vi "Corrupt DLC.vi"(8 "error in (no error)":errorcluster, 9 "Engine Run-Time Data Cluster In":T1 {"Compiled Data"."Corruption Info DUT_Network"."Frame Infos Array"."CRC Index" min=-7 max=7; "Compiled Data"."Corruption Info DUT_Network"."Frame Infos Array"."DLC Length  Corruption Index" min=-8 max=8; "Compiled Data"."Corruption Info Network_DUT"."Frame Infos Array"."CRC Index" min=-7 max=7; "Compiled Data"."Corruption Info Network_DUT"."Frame Infos Array"."DLC Length  Corruption Index" min=-8 max=8; "Specified Channel Ref List Out" format="%.0x"; "Specified Channel Ref List In" format="%.0x"}, 10 "Frame Infos":T6 {"CRC Index" min=-7 max=7; "DLC Length  Corruption Index" min=-8 max=8}, 11 "CAN frame in":T8 {"payload" format="%x"; "timestamp" format="%<%.7X\n%x>T"; "type" items=["CAN Data"=0, "CAN Remote"=1, "CAN Bus Error"=2, "CAN 2.0 Data"=8, "CAN FD Data"=16, "CAN FD+BRS Data"=24, "J1939 Data"=192, "Delay"=224, "Log Trigger"=225, "Start Trigger"=226]; "identifier" format="%x"}) -> (0 "error out":errorcluster, 3 "CAN frame out":T8 {"payload" format="%x"; "timestamp" format="%<%.7X\n%x>T"; "type" items=["CAN Data"=0, "CAN Remote"=1, "CAN Bus Error"=2, "CAN 2.0 Data"=8, "CAN FD Data"=16, "CAN FD+BRS Data"=24, "J1939 Data"=192, "Delay"=224, "Log Trigger"=225, "Start Trigger"=226]; "identifier" format="%x"})   [LabVIEW 2018, in "CAN Gateway Engine.lvlib"]
uses:
  CAN Gateway Engine.lvlib
  <vilib>/xnet/xnet.llb/XNET Frame CAN.ctl
  <vilib>/xnet/xnet.llb/XNET Frame Type CAN.ctl
  Shared/CTLs/Frame.ctl
  Shared/CTLs/Signal_Data_Trigger.ctl
  Shared/CTLs/Runtime engine Data.ctl
  <vilib>/NI Veristand/Custom Device API/Custom Device Engine Event Ref.ctl
  <vilib>/NI Veristand/Custom Device API/Custom Device Item Ref.ctl
  Shared/CTLs/Compiled Data.ctl
  Shared/CTLs/Corruption Info.ctl
  Shared/CAN Gateway Shared.lvlib
  <vilib>/NI Veristand/Custom Device API/Custom Device API.lvlib
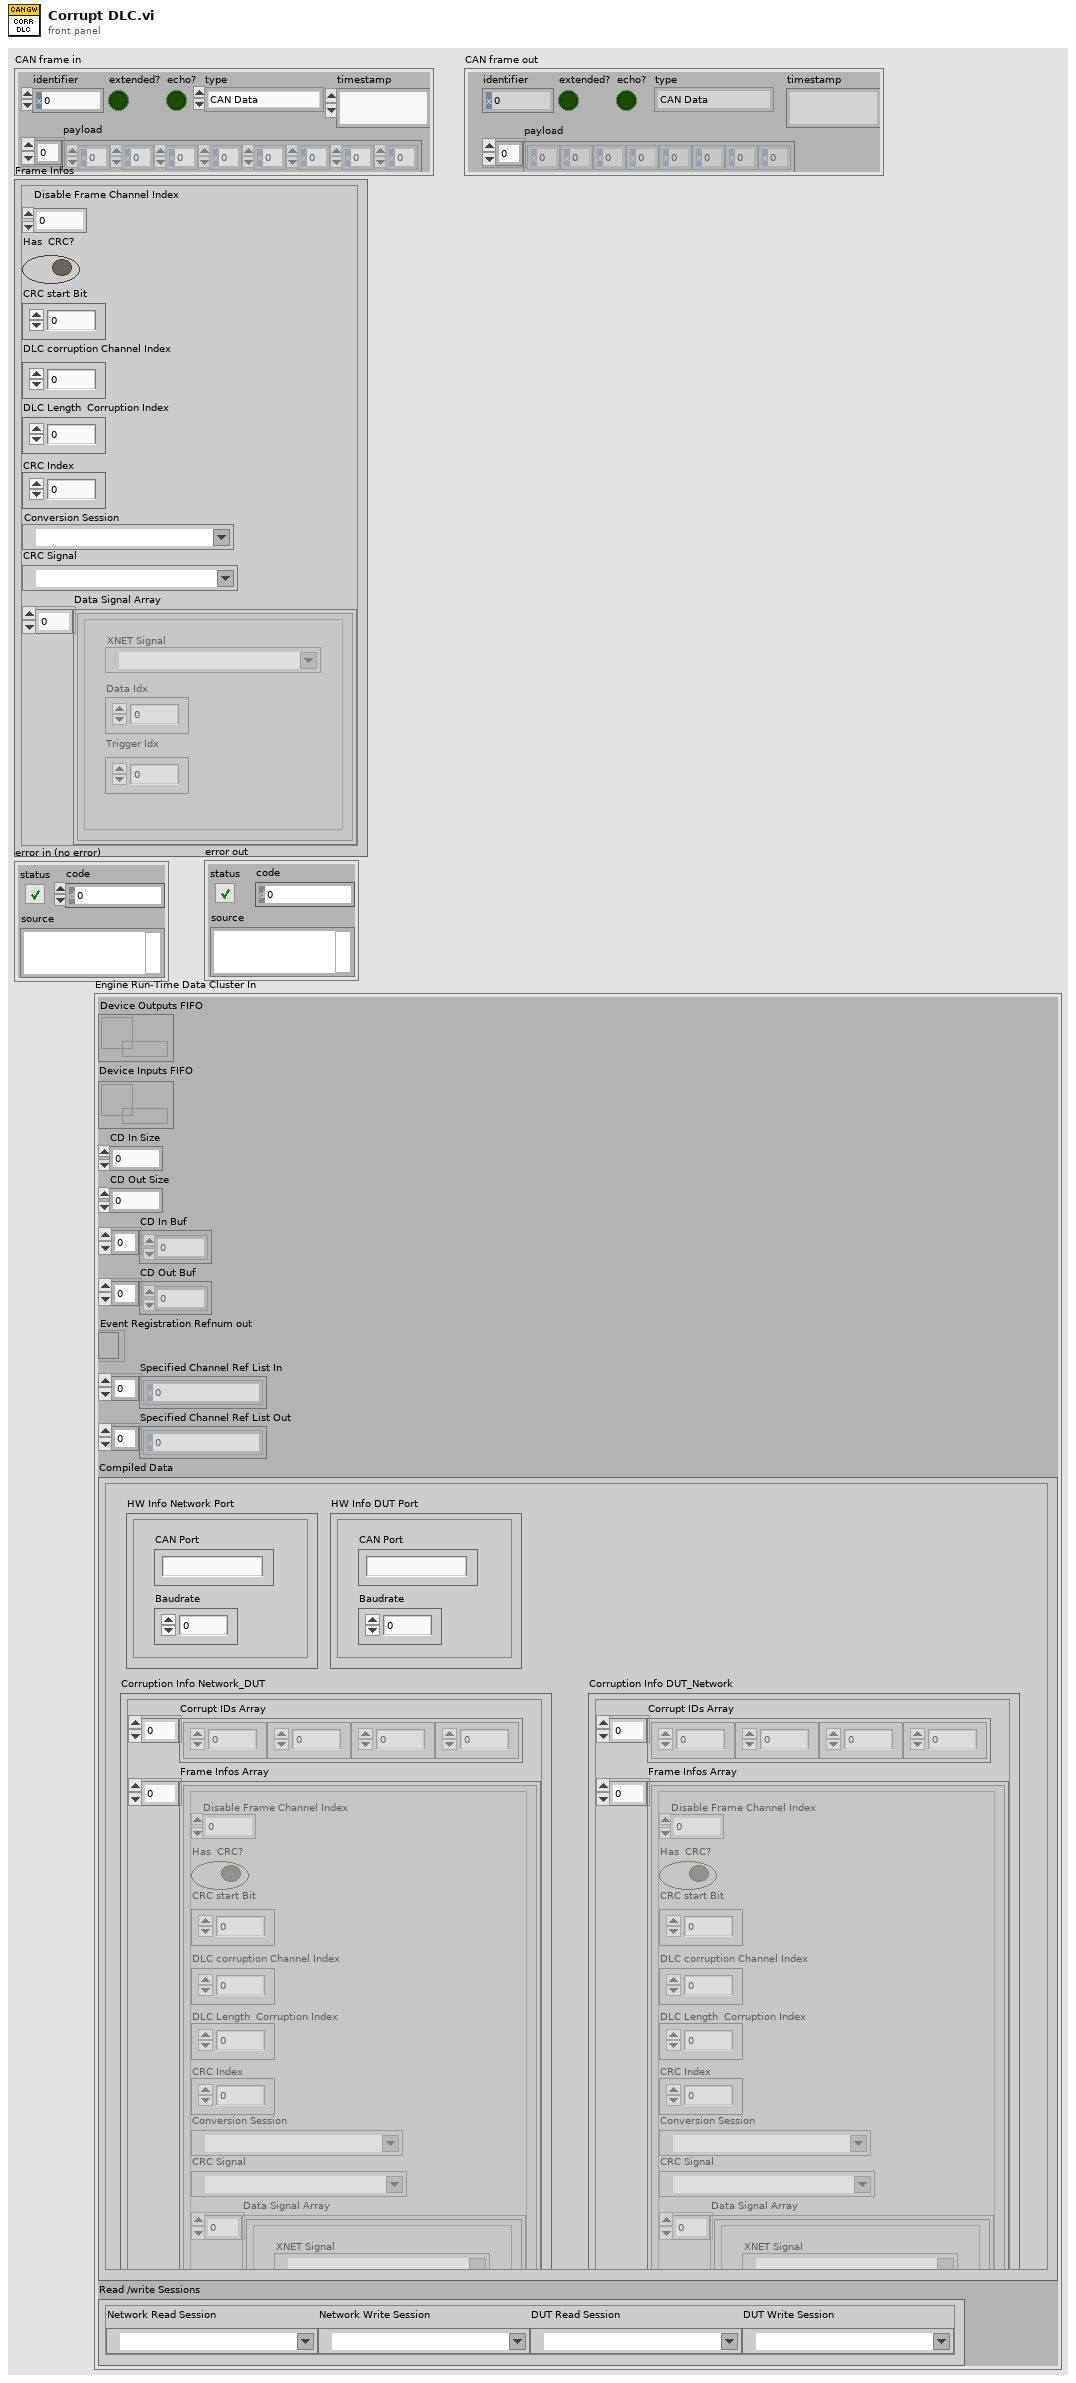
[diagram p1: front panel]
types:
  T1 = typedef "CAN Gateway Engine.lvlib/Runtime engine Data.ctl" = cluster{"Device Outputs FIFO":refnum<k33>, "Device Inputs FIFO":refnum<k33>, "CD In Size":i32, "CD Out Size":i32, "CD In Buf":dbl[], "CD Out Buf":dbl[], "Event Registration Refnum out":T2, "Specified Channel Ref List In":T3[], "Specified Channel Ref List Out":T3[], "Compiled Data":T4, "Read /write Sessions":cluster{"Network Read Session":refnum<k21>, "Network Write Session":refnum<k21>, "DUT Read Session":refnum<k21>, "DUT Write Session":refnum<k21>}}
  T2 = typedef "Custom Device API.lvlib/Custom Device Engine Event Ref.ctl" = refnum<event-registration>
  T3 = typedef "Custom Device API.lvlib/Custom Device Item Ref.ctl" = u64
  T4 = typedef "CAN Gateway Shared.lvlib/Compiled Data.ctl" = cluster{"HW Info Network Port":cluster{"CAN Port":string, "Baudrate":u64}, "HW Info DUT Port":cluster{"CAN Port":string, "Baudrate":u64}, "Corruption Info Network_DUT":T5, "Corruption Info DUT_Network":T5}
  T5 = typedef "CAN Gateway Shared.lvlib/Corruption Info.ctl" = cluster{"Corrupt IDs Array":u32[], "Frame Infos Array":T6[]}
  T6 = typedef "CAN Gateway Shared.lvlib/Frame.ctl" = cluster{"Disable Frame Channel Index":i32, "Has  CRC?":bool, "CRC start Bit":u32, "DLC corruption Channel Index":i32, "DLC Length  Corruption Index":i32, "CRC Index":i32, "Conversion Session":refnum<k21>, "CRC Signal":refnum<k21>, "Data Signal Array":T7[]}
  T7 = typedef "CAN Gateway Shared.lvlib/Signal_Data_Trigger.ctl" = cluster{"XNET Signal":refnum<k21>, "Data Idx":u32, "Trigger Idx":u32}
  T8 = typedef "XNET Frame CAN.ctl" = cluster{"timestamp":timestamp, "payload":u8[], "identifier":u32, "type":T9, "extended?":bool, "echo?":bool}
  T9 = typedef "XNET Frame Type CAN.ctl" = u8
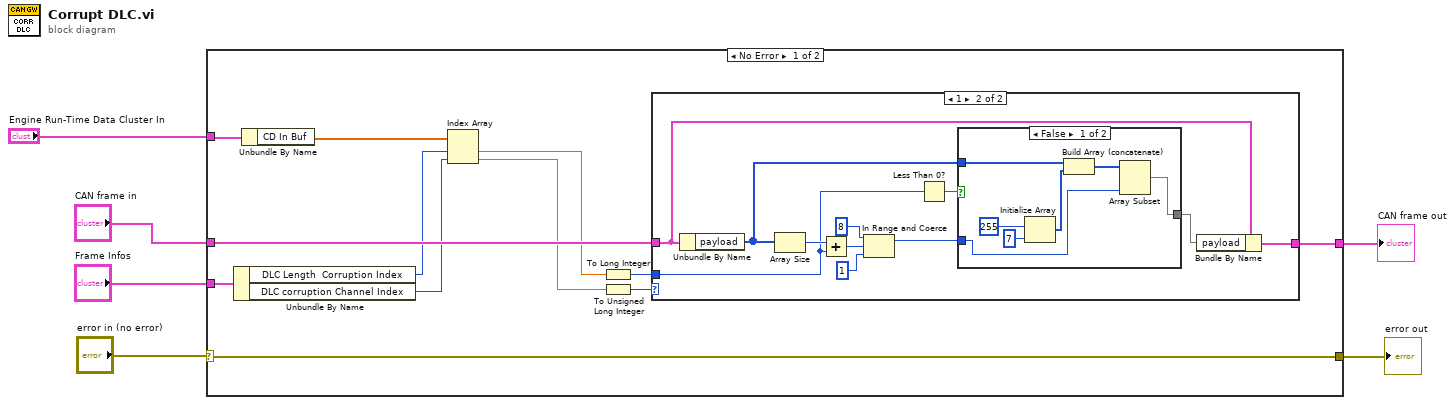
[diagram p0: block diagram]
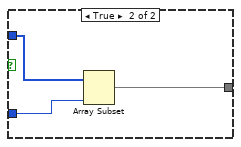
[diagram p3: hidden frame]
diagram:
  n1 = case shown="No Error" "error in (no error)" {
    selector: "error in (no error)" -> [w15 w41]
    tunnel: "CAN frame in" -> [w18 w42]
    tunnel: [w17 w42] -> w5
    tunnel: "Frame Infos" -> [w16 _]
    tunnel: [w15 w41] -> w2
    tunnel: "Engine Run-Time Data Cluster In" -> [w14 _]
    frame No Error {
      n2 = Unbundle By Name(w16) -> ("DLC Length  Corruption Index"=w12:i32, "DLC corruption Channel Index"=w11:i32)
      n3 = Unbundle By Name(w14) -> ("CD In Buf"=w13:dbl[])
      n4 = Index Array(array=w13, index #1=w12, index #2=w11) -> (element #1=w10:dbl, element #2=w9:dbl)
      n5 = To Long Integer(number=w10) -> (32bit integer=w7:i32)
      n6 = To Unsigned Long Integer(number=w9) -> (unsigned 32bit integer=w8:u32)
      n7 = case shown="1" w8 {
        tunnel: w18 -> [w19 w26]
        tunnel: [w19 w24] -> w17
        tunnel: w7 -> [_ w20]
        frame 0, Default {
        }
        frame 1 {
          n8 = Unbundle By Name(w26) -> ("payload"=w27:u8[])
          n9 = Array Size(array=w27) -> (size(s)=w23:i32)
          n10 = Add(x=w23, y=w20) -> (x+y=w30:i32)
          n11 = In Range and Coerce(upper limit=8, x=w30, lower limit=1) -> (coerced(x)=w22:i32)  [unwired: 1 out]
          n12 = Less Than 0?(x=w20) -> (x < 0?=w21:bool)
          n13 = case shown="False" w21 {
            tunnel: w27 -> [w34 w40]
            tunnel: [w31 w39] -> w25
            tunnel: w22 -> [w32 w38]
            frame False {
              n14 = Initialize Array(u8 255, 7 ("dimension size")) -> (w35:u8[])
              n15 = Build Array (concatenate)(w34, w35) -> (w33:u8[])
              n16 = Array Subset(array=w33, length=w32) -> (w31:u8[])  [unwired: 1 in]
            }
            frame True {
              n17 = Array Subset(array=w40, length=w38) -> (w39:u8[])  [unwired: 1 in]
            }
          }
          n18 = Bundle By Name(cluster=w26, "payload"=w25) -> (w24:T8)
        }
      }
    }
    frame Error {
    }
  }
  "CAN frame out" <- w5
  "error out" <- w2
